vi "Kostka.vi"() -> ()   [LabVIEW 2022 SP3]
uses:
  <vilib>/numeric/Random Number (Range) I64.vi
  <vilib>/numeric/sub_Random U32.vi
panel:
  in  "?":bool
  in  "?":bool
  out "?":bool
  out "?":bool
  out "?":bool
  out "?":bool
  out "?":bool
  out "?":bool
  out "?":bool
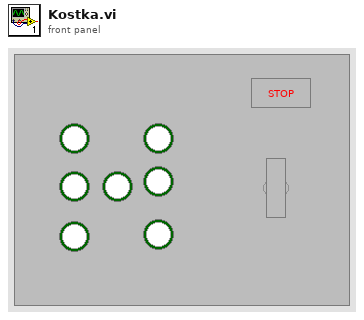
[diagram p1: front panel]
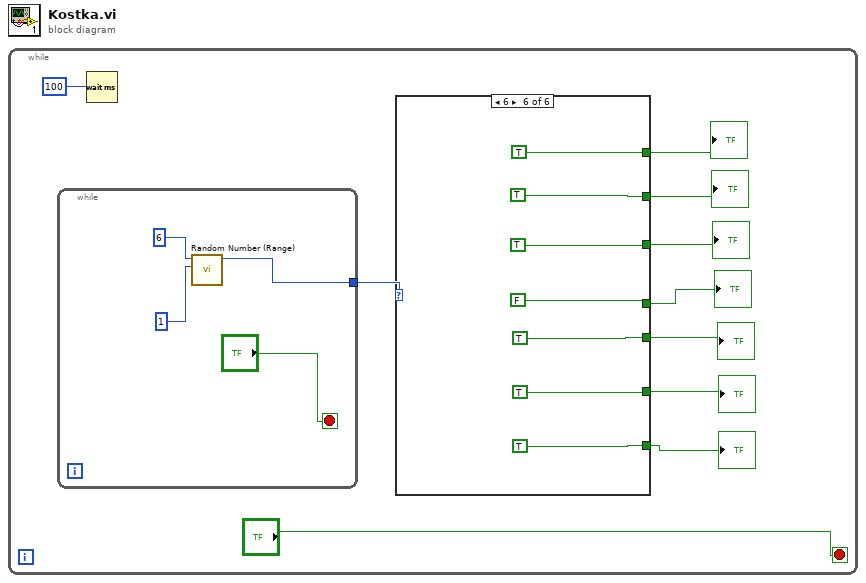
[diagram p0: block diagram]
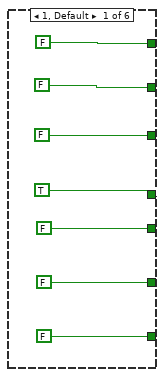
[diagram p2: hidden frame]
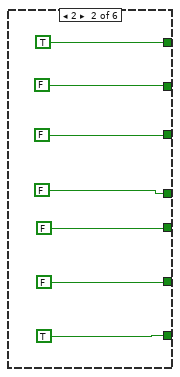
[diagram p3: hidden frame]
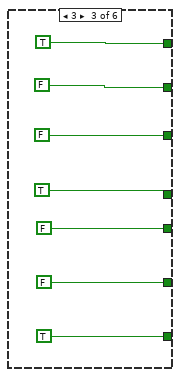
[diagram p4: hidden frame]
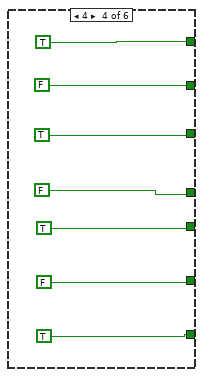
[diagram p5: hidden frame]
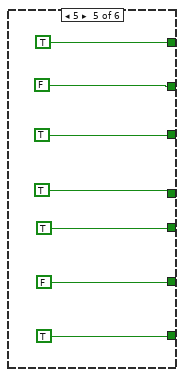
[diagram p6: hidden frame]
diagram:
  n1 = while {
    stop <- "?" stop-if-true
    n2 = while {
      tunnel: [w54] -> w10
      stop <- "?" stop-if-true
      n3 = call-poly <vilib>:"Random Number (Range).vi"("lower bound (-100)"=1, "upper bound (100)"=6) -> ("number"=w54:i64)  [unwired: 9 in]
    }
    n4 = Wait (ms)(milliseconds to wait=100) -> ()  [unwired: 1 out]
    n5 = case shown="6" w10 {
      tunnel: [TRUE FALSE TRUE FALSE TRUE FALSE] -> w9
      tunnel: [FALSE TRUE TRUE TRUE TRUE TRUE] -> w8
      tunnel: [FALSE FALSE FALSE FALSE FALSE TRUE] -> w7
      tunnel: [FALSE FALSE FALSE TRUE TRUE TRUE] -> w6
      tunnel: [FALSE FALSE FALSE TRUE TRUE TRUE] -> w5
      tunnel: [FALSE FALSE FALSE FALSE FALSE TRUE] -> w4
      tunnel: [FALSE TRUE TRUE TRUE TRUE TRUE] -> w3
      frame 1, Default {
      }
      frame 2 {
      }
      frame 3 {
      }
      frame 4 {
      }
      frame 5 {
      }
      frame 6 {
      }
    }
    "?" <- w3
    "?" <- w4
    "?" <- w5
    "?" <- w9
    "?" <- w6
    "?" <- w7
    "?" <- w8
  }
